vi "Boolean Delay 2.vi"(2 "Input":bool, 3 "Delay (ms)":dbl) -> (0 "Output":bool)   [LabVIEW 2015]
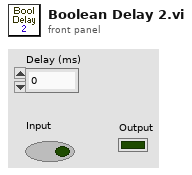
[diagram p1: front panel]
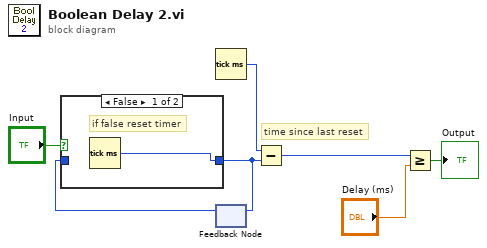
[diagram p0: block diagram]
diagram:
  # "time since last reset"
  n1 = Tick Count (ms)() -> (millisecond timer value=w7:u32)
  n2 = feedback #1() -> (w6:u32)  [unwired: 1 in]
  n3 = case shown="False" "Input" {
    tunnel: [w8 w9] -> w5
    tunnel: w6 -> [_ w9]
    frame False {
      # "if false reset timer"
      n4 = Tick Count (ms)() -> (millisecond timer value=w8:u32)
    }
    frame True {
      # "if true don't reset timer"
    }
  }
  n5 = feedback-in #1(w5) -> ()
  n6 = Subtract(x=w7, y=w5) -> (x-y=w3:u32)
  n7 = Greater Or Equal?(x=w3, y="Delay (ms)") -> (x >= y?=→"Output":bool)
